vi "_CSMObj-Remove Chain Node.vi"(8 "Error In":errorcluster caption="error in (no error)", 10 "Requested Name":string, 11 "CSMObj In":T1={"info"={"Module Name"="", "Requested Name"="", "Group Name"="", "Mode"=enum."Stand Alone", "Allowed Messages"=[]}, "Refs"={"WatchDogQ"=refnum, "CSMDataDVR"=refnum, "Queue"={"HPriorityQ"=refnum, "LowPriorityQ"=refnum}, "GroupDataDVR"=refnum, "TagMap"=refnum, "ExitEvent"=refnum, "NewStateEvent"=refnum, "StatusEvent"=refnum, "InterruptEvent"=refnum}}) -> (0 "error out":errorcluster, 3 "CSMObj Out":T1={"info"={"Module Name"="", "Requested Name"="", "Group Name"="", "Mode"=enum."Stand Alone", "Allowed Messages"=[]}, "Refs"={"WatchDogQ"=refnum, "CSMDataDVR"=refnum, "Queue"={"HPriorityQ"=refnum, "LowPriorityQ"=refnum}, "GroupDataDVR"=refnum, "TagMap"=refnum, "ExitEvent"=refnum, "NewStateEvent"=refnum, "StatusEvent"=refnum, "InterruptEvent"=refnum}})   [LabVIEW 2017, in "Communicable State Machine.lvlib"]
uses:
  Communicable State Machine.lvlib
  _CSMObj.ctl
  _CSMObj-Info.ctl
  Typedef/_CSM_MODE.ctl
  _CSMObj-Refs.ctl
  _CSMObj-Data.ctl
  Priority Queue/Priority Queue.ctl
  Typedef/_Cross CSM State Data.ctl
  Typedef/_CSM_MSG_TYPE.ctl
  Typedef/_Cross CSM State Response.ctl
  Typedef/_CSM_Response Source Message.ctl
  Priority Queue/def-Data(LowPRI-Q).ctl
  _CSMObj-ModeData.ctl
  Typedef/_CSM Status Change Event Data.ctl
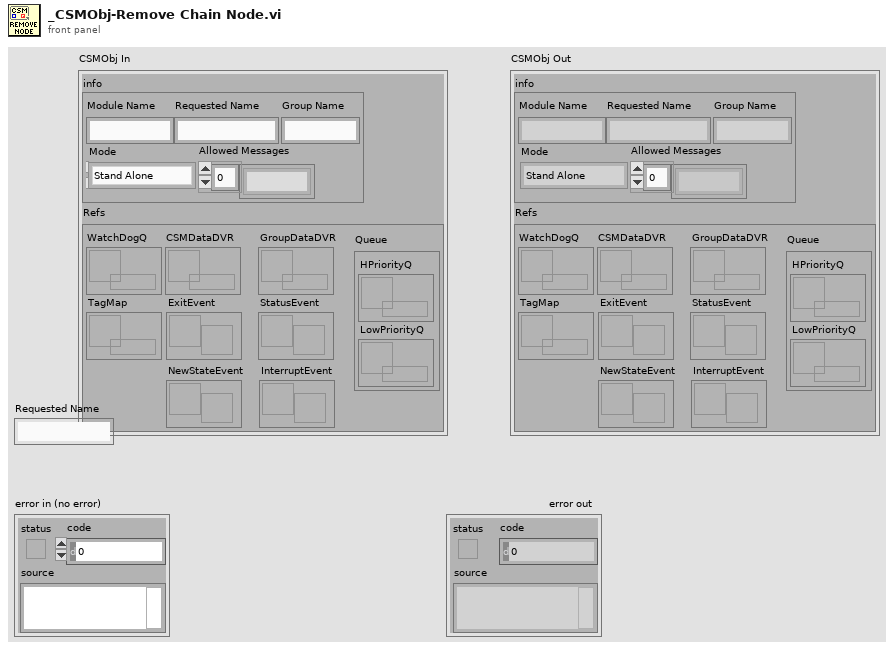
[diagram p1: front panel]
types:
  T1 = typedef "Communicable State Machine.lvlib/_CSMObj.ctl" = cluster{"info":T2, "Refs":T4}
  T2 = typedef "Communicable State Machine.lvlib/_CSMObj-Info.ctl" = cluster{"Module Name":string, "Requested Name":string, "Group Name":string, "Mode":T3, "Allowed Messages":string[]}
  T3 = typedef "Communicable State Machine.lvlib/_CSM_MODE.ctl" = enum16{"Not Exist", "Stand Alone", "CSM", "Worker", "Worker Agent", "Chain Node", "Chain"}
  T4 = typedef "Communicable State Machine.lvlib/_CSMObj-Refs.ctl" = cluster{"WatchDogQ":refnum<queue>, "CSMDataDVR":refnum<data-value>, "Queue":T5, "GroupDataDVR":refnum<data-value>, "TagMap":refnum<data-value>, "ExitEvent":refnum<user-event>, "NewStateEvent":refnum<user-event>, "StatusEvent":refnum<user-event>, "InterruptEvent":refnum<user-event>}
  T5 = typedef "Communicable State Machine.lvlib/Priority Queue.ctl" = cluster{"HPriorityQ":refnum<queue>, "LowPriorityQ":refnum<queue>}
  T6 = typedef "Communicable State Machine.lvlib/_CSMObj-ModeData.ctl" = cluster{"CSMDataDVR":refnum<data-value>[], "PriorityQueues":T5[], "Messages of Chain Nodes":cluster{"Module Name":string, "Allowed Messages":string[]}[], "Chain Message Mapping Map":variant, "SharedRegistryRules":string[]}
  T7 = cluster{"Module Name":string, "Allowed Messages":string[]}[]
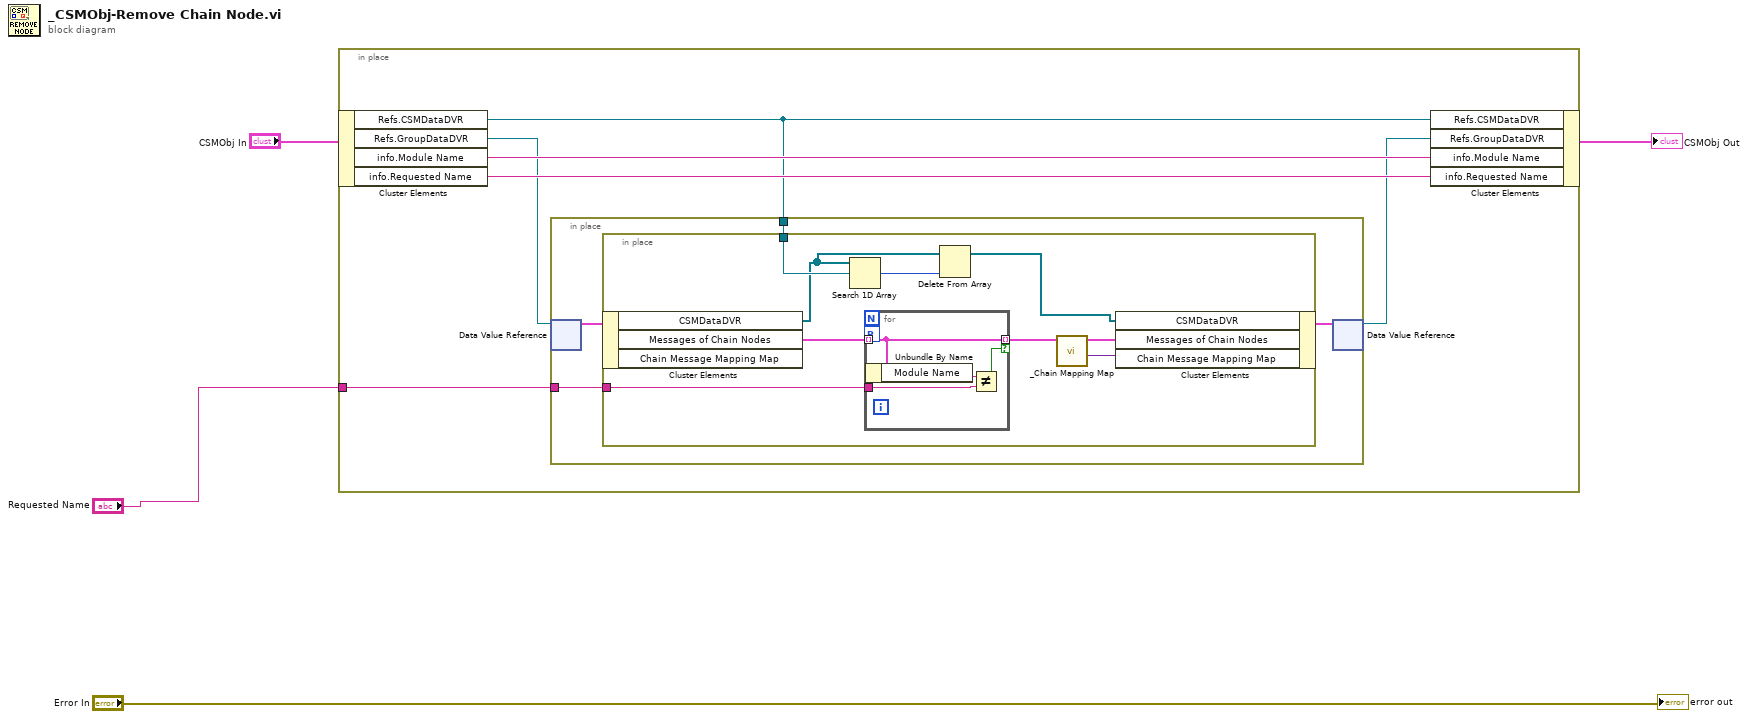
[diagram p0: block diagram]
diagram:
  n1 = in-place "In Place Element Structure" {
    in-place-border: "Requested Name" -> [w6]
    n2 = in-place-cluster #1("CSMObj In") -> ("Refs.CSMDataDVR"=w5:refnum<data-value>, "Refs.GroupDataDVR"=w8:refnum<data-value>, "info.Module Name"=w10:string, "info.Requested Name"=w9:string)
    n3 = in-place {
      in-place-border: w6 -> [w12]
      in-place-border: w5 -> [w11]
      n4 = in-place-dvr #2(w8) -> (w14:T6)  [unwired: 1 out]
      n5 = in-place {
        in-place-border: w12 -> [w20]
        in-place-border: w11 -> [w18]
        n6 = in-place-cluster #3(w14) -> ("CSMDataDVR"=w16:refnum<data-value>[], "Messages of Chain Nodes"=w21:T7)  [unwired: 1 out]
        n7 = Search 1D Array(1D array=w16, element=w18) -> (index of element=w17:i32)  [unwired: 1 in]
        n8 = for {
          tunnel: w21 -> [w27] mode=indexing
          tunnel: [w27] -> w19 mode=indexing if=w24
          tunnel: w20 -> [w25]
          workers-P: _ -> [_]
          n9 = Unbundle By Name(w27) -> ("Module Name"=w26:string)
          n10 = Not Equal?(x=w26, y=w25) -> (x != y?=w24:bool)
        }
        n11 = Delete From Array(array=w16, index=w17) -> (array with subset deleted=w15:refnum<data-value>[])  [unwired: 1 in, 1 out]
        n12 = call "_Chain Mapping Map.vi"("Messages of Chain Nodes"=w19) -> ("Variant"=w22:variant, "Messages of Chain Nodes (Dup)"=w23:T7)  [unwired: 9 in]
        n13 = in-place-cluster #3("CSMDataDVR"=w15, "Messages of Chain Nodes"=w23, "Chain Message Mapping Map"=w22) -> (w13:T6)
      }
      n14 = in-place-dvr #2(w13) -> (w7:refnum<data-value>)  [unwired: 1 out]
    }
    n15 = in-place-cluster #1("Refs.CSMDataDVR"=w5, "Refs.GroupDataDVR"=w7, "info.Module Name"=w10, "info.Requested Name"=w9) -> (→"CSMObj Out":T1)
  }
  "error out" <- "Error In"
